vi "Upload File.vi"(4 "attributes":refnum<class "File Attributes.lvclass">, 6 "timeout (ms)":i32=30000, 8 "error in":errorcluster, 9 "remote path":string, 10 "local path":path, 11 "session in":refnum<class "Session.lvclass">) -> (0 "error out":errorcluster, 3 "session out":refnum<class "Session.lvclass">)   [LabVIEW 2020, in "NI_SFTP.lvlib"]
doc: "Creates a new remote file, initialized with the contents of a local file."
uses:
  <vilib>/net/SFTP/NI_SFTP.lvlib
  <vilib>/net/SFTP/Session/Session.lvclass
  <vilib>/net/SFTP/File Attributes/File Attributes.lvclass
  <vilib>/net/SFTP/API/Support/Upload/File/File Upload Controller.lvclass
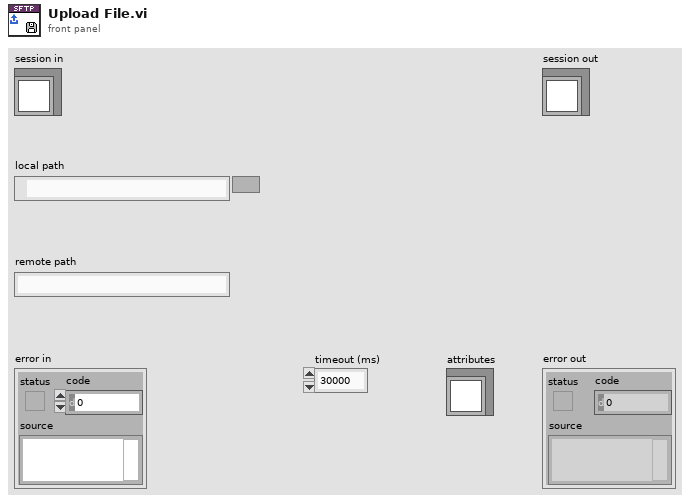
[diagram p1: front panel]
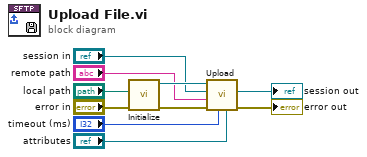
[diagram p0: block diagram]
diagram:
  n1 = call <vilib>:"Initialize.vi"("error in (no error)"="error in", "local path"="local path") -> ("error out"=w7:errorcluster, "File Upload Controller out"=w8:refnum<class "File Upload Controller.lvclass">)  [unwired: 8 in]
  n2 = call-dynamic "Upload.vi"("attributes"="attributes", "timeout (ms)"="timeout (ms)", "error in"=w7, "remote path"="remote path", "session in"="session in", "NI_SFTP.lvlib:Generic Upload Controller.lvclass"=w8) -> ("error out"=→"error out":errorcluster, "session out"=→"session out":refnum<class "Session.lvclass">)  [unwired: 3 in, 1 out]
